vi "Test Speed.vi"() -> ()   [LabVIEW 2024]
panel:
  out "XY Graph":cluster{dbl[], dbl[]}[](graph)
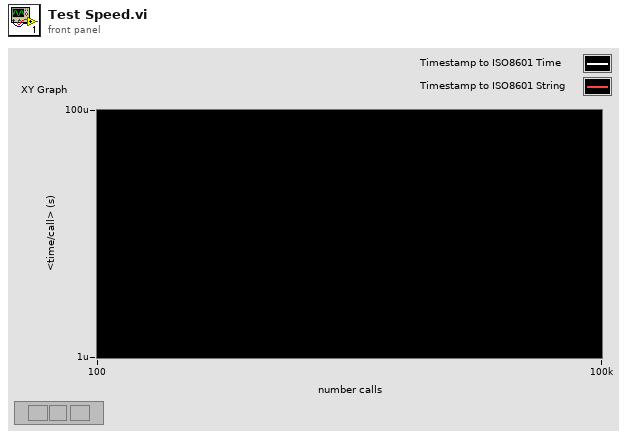
[diagram p1: front panel]
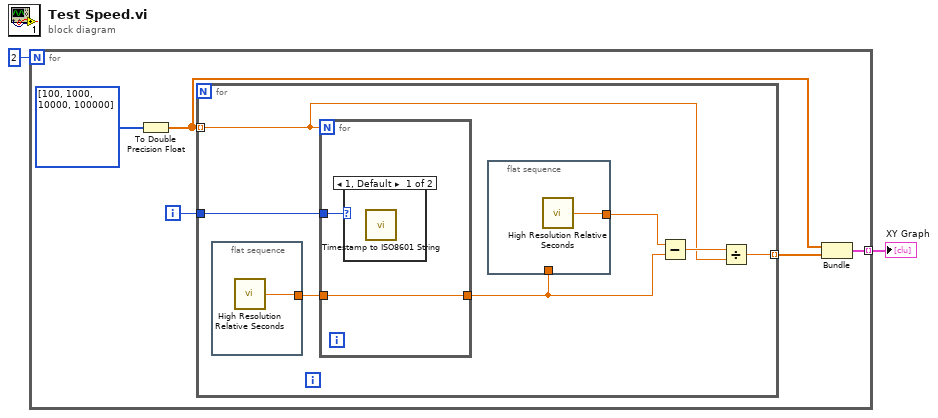
[diagram p0: block diagram]
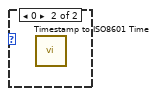
[diagram p2: hidden frame]
diagram:
  n1 = for {
    N: 2 -> [_]
    tunnel: [w4] -> w1 mode=indexing
    i -> [w3]
    n2 = To Double Precision Float(number=i32[] [100, 1000, 10000, 100000] ("Array")) -> (double precision float=w5:dbl[])
    n3 = for {
      tunnel: w5 -> [w12] mode=indexing
      tunnel: [w11] -> w6 mode=indexing
      tunnel: w3 -> [w8]
      n4 = flat-sequence {
        tunnel: [w15] -> w13
        frame #0 {
          n5 = call <vilib>:"High Resolution Relative Seconds.vi"() -> ("relative seconds"=w15:dbl)
        }
      }
      n6 = for {
        N: w12 -> [_]
        tunnel: w13 -> [w18]
        tunnel: [w18] -> w9
        tunnel: w8 -> [w17]
        n7 = case shown="1, Default" w17 {
          frame 1, Default {
            n8 = call "Timestamp to ISO8601 String.vi"() -> ()  [unwired: 11 in, 1 out]
          }
          frame 0 {
            n9 = call "Timestamp to ISO8601 Time.vi"() -> ()  [unwired: 11 in, 1 out]
          }
        }
      }
      n10 = flat-sequence {
        tunnel: [w16] -> w10
        tunnel: w9 -> [_]
        frame #0 {
          n11 = call <vilib>:"High Resolution Relative Seconds.vi"() -> ("relative seconds"=w16:dbl)
        }
      }
      n12 = Subtract(x=w10, y=w9) -> (x-y=w14:dbl)
      n13 = Divide(x=w14, y=w12) -> (x/y=w11:dbl)
    }
    n14 = Bundle(w5, w6) -> (w4:cluster{dbl[], dbl[]})  [unwired: 1 in]
  }
  "XY Graph" <- w1
